vi "Image Thresholding.vi"() -> ()   [LabVIEW 2018]
uses:
  <vilib>/vision/NI_Vision_Development_Module.lvlib
panel:
  in  "Stop Button":bool
  out "Calibrated":bool
  in  "Threshold Range":cluster{sgl, sgl}(slide)={0.0, 255.0} scale=0.0..255.0
  out "Grayscale Intensity Histogram":u32[](graph)
  out "Camera Image":T1(plugin-control)
  out "Processed Image":T1(plugin-control)
  # "Mechatronic Actuators Board"
  # "Image Thresholding"
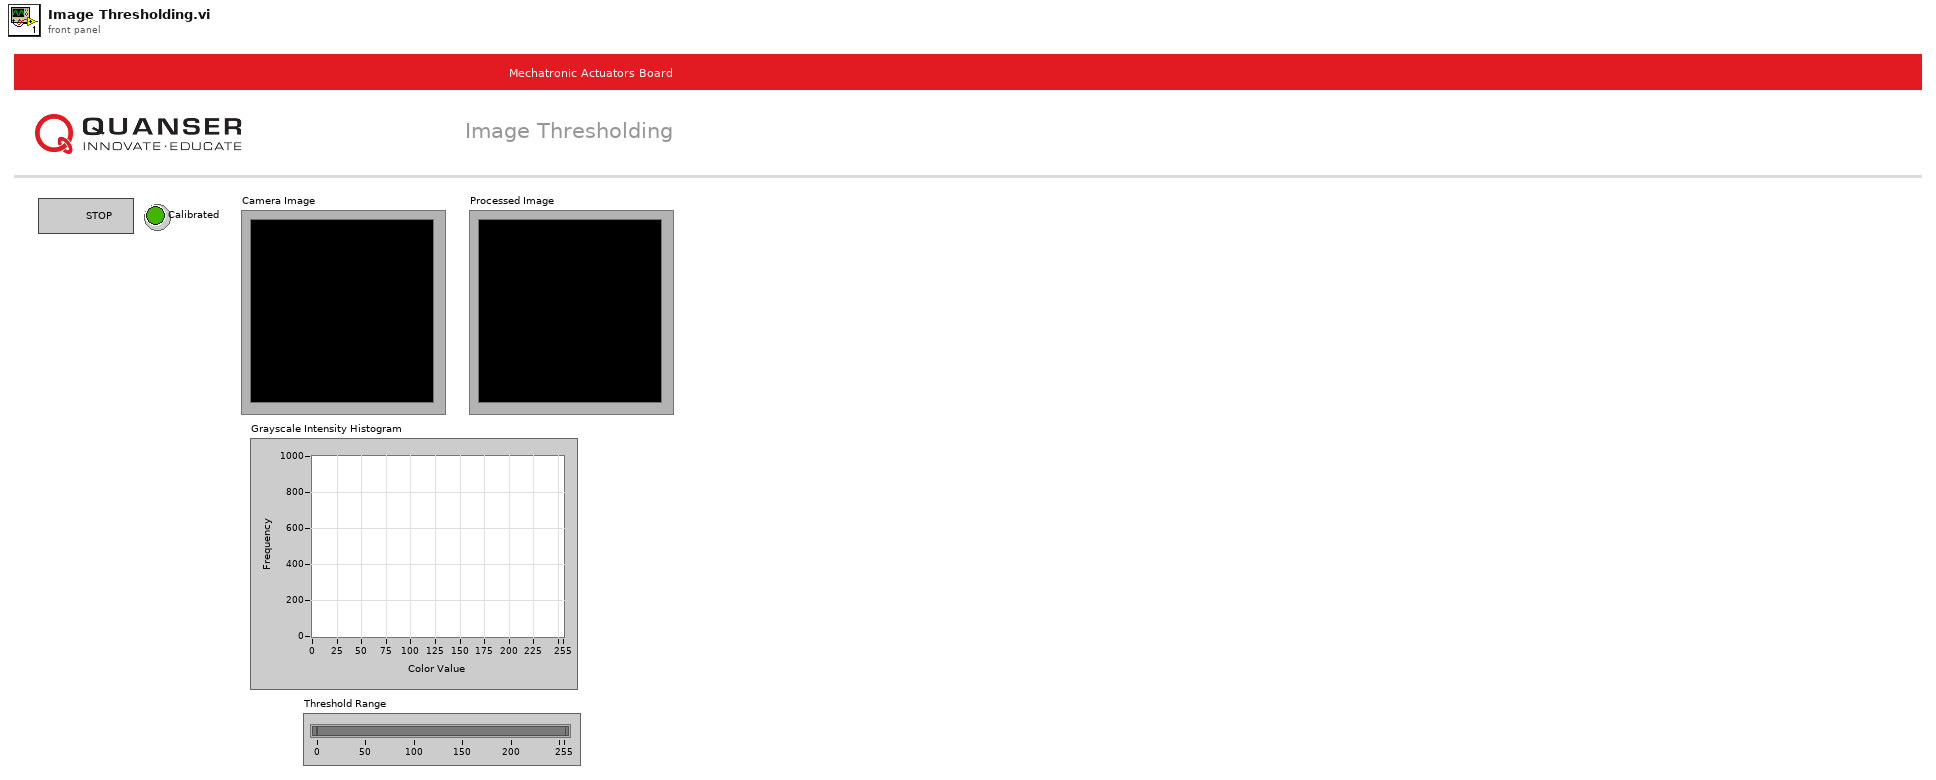
[diagram p1: front panel]
types:
  T1 = typedef "IMAQ Image.ctl" = refnum<image>
  T2 = typedef "QNET MS IO Cluster.ctl" = cluster{"Error":errorcluster, "Encoder Calibration Values":i32[], "Update Calibration":bool, "JPEG Resolutions":u16, "Raw Resolutions":u16, "Image Mode":enum16{"RAW RGB", "RAW Gray Scale", "JPEG"}, "FPGA Ref":refnum<k20>}
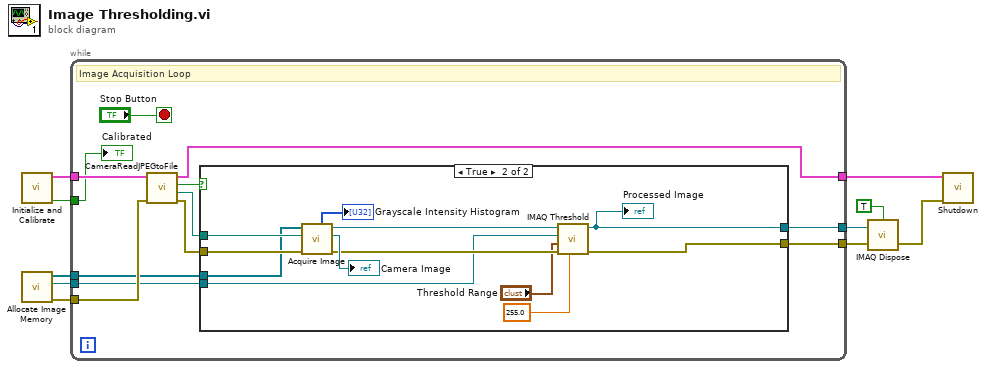
[diagram p0: block diagram]
diagram:
  n1 = call "Initialize and Calibrate.vi"() -> ("Calibrated"=w5:bool, "IO Cluster"=w6:T2)  [unwired: 10 in]
  n2 = call "Allocate Image Memory.vi"() -> ("error out"=w4:errorcluster, "HSL Threshold"=w1:T1, "Acquisition Memory"=w2:T1[])  [unwired: 6 in, 3 out]
  n3 = while {
    tunnel: w6 -> [w22]
    tunnel: [w11] -> w7
    tunnel: [w21] -> w9
    tunnel: [w19] -> w8
    tunnel: w5 -> [w16]
    tunnel: w4 -> [w14]
    tunnel: w2 -> [w12]
    tunnel: w1 -> [w13]
    stop <- "Stop Button" stop-if-true
    # "Image Acquisition Loop"
    n4 = call "CameraReadJPEGtoFile.vi"("error in"=w14, "IO Cluster In"=w22) -> ("Error Out"=w20:errorcluster, "Image File"=w15:path, "New Image Data"=w18:bool, "IO Cluster Out"=w11:T2)  [unwired: 6 in]
    n5 = case shown="True" w18 {
      tunnel: [w24 w30] -> w21
      tunnel: w15 -> [_ w35]
      tunnel: w20 -> [w24 w36]
      tunnel: [w23 w28] -> w19
      tunnel: w13 -> [w23 w26]
      tunnel: w12 -> [_ w27]
      frame False {
      }
      frame True {
        n6 = call "Acquire Image.vi"("Error In"=w36, "File Path"=w35, "Acquisition Memory"=w27) -> ("Error Out"=w31:errorcluster, "HSL Image"=→"Camera Image":T1, "Pre-processed Image"=w32:T1, "histogram"=→"Grayscale Intensity Histogram":u32[])  [unwired: 4 in, 1 out]
        n7 = call "IMAQ Threshold"("Replace Value"=sgl 255.0, "error in (no error)"=w31, "Range"="Threshold Range", "Image Dst"=w26, "Image Src"=w32) -> ("error out"=w30:errorcluster, "Image Dst Out"=w28:T1)  [unwired: 5 in]
        "Processed Image" <- w28
      }
    }
    "Calibrated" <- w16
  }
  n8 = call "IMAQ Dispose"("All Images? (No)"=TRUE, "Image"=w8, "error in (no error)"=w9) -> ("error out"=w10:errorcluster)  [unwired: 3 in]
  n9 = call "Shutdown.vi"("Image Processing Loop"=w10, "IO Cluster In"=w7) -> ()  [unwired: 9 in, 1 out]
